vi "About WTI.vi"(0 "Description and Version":string, 1 "Designers":string[](array[string]), 2 "Contact Information In":string) -> ()   [LabVIEW 2019]
panel:
  in  "Exit":bool
  out "Project Description":string
  out "Designers:":string
  out "Contact Information:":string
  in  "SHDocVw.IWebBrowser2":refnum<k7>(container)
  # "System Developed with National Instruments LabVIEW"
  # "Copyright 2001 Wineman Technology Inc."
  # "Click Screen or Press Enter To Continue"
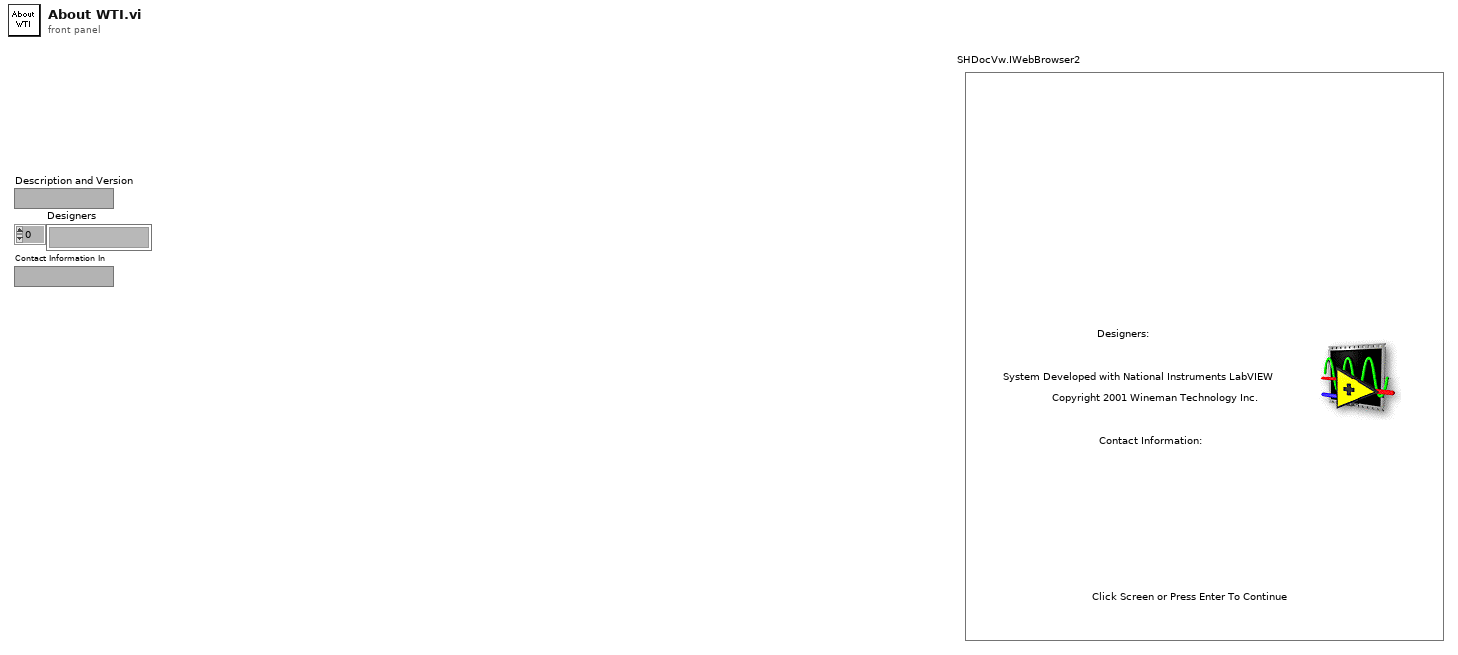
[diagram p1: front panel]
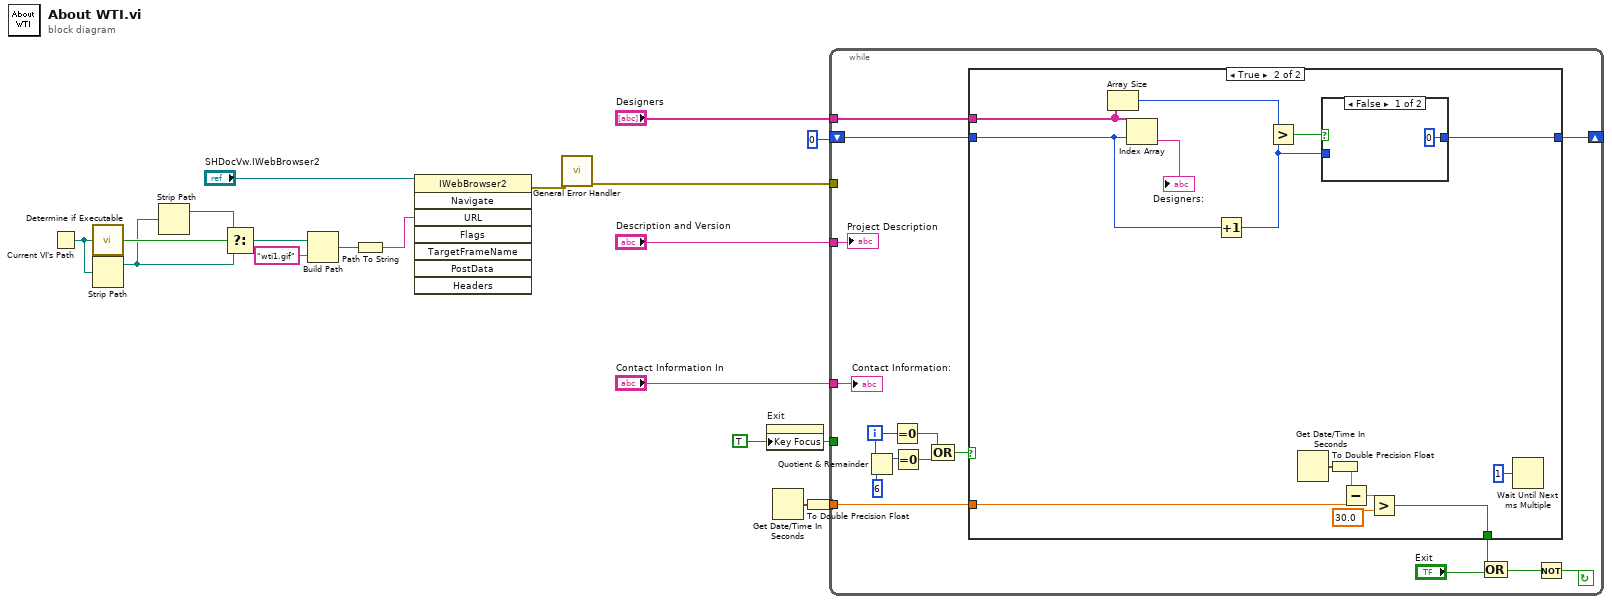
[diagram p0: block diagram]
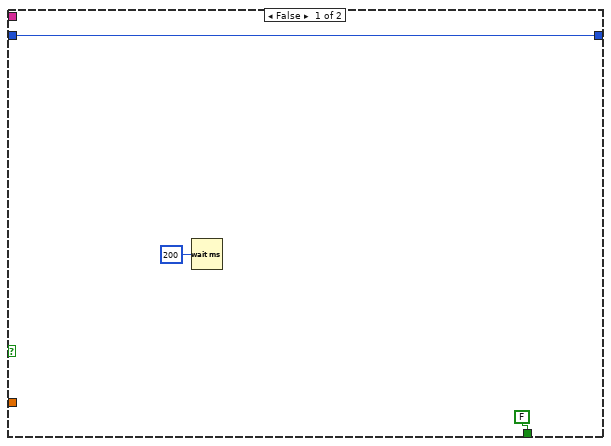
[diagram p2: hidden frame]
diagram:
  w13 = TRUE ("Key Focus")
  n1 = Current VI's Path() -> (path=w5:path)
  n2 = call "Determine if Executable.vi"("Path"=w5) -> ("EXE?"=w6:bool)
  n3 = Strip Path(path=w5) -> (stripped path=w4:path)  [unwired: 1 out]
  n4 = Strip Path(path=w4) -> (stripped path=w3:path)  [unwired: 1 out]
  n5 = Select(t=w3, s=w6, f=w4) -> (s? t:f=w2:path)
  n6 = Build Path(base path=w2, name or relative path="wti1.gif") -> (appended path=w11:path)
  n7 = Path To String(path=w11) -> (string=w10:string)
  n8 = invoke class="IWebBrowser2" method="Navigate"(reference="SHDocVw.IWebBrowser2", "URL"=w10) -> (error out=w9:errorcluster)  [unwired: 6 in, 7 out]
  n9 = call <vilib>:"General Error Handler.vi"("error in (no error)"=w9) -> ("error out"=w7:errorcluster)  [unwired: 10 in, 4 out]
  n10 = property on="Exit" class="Bool"("Key Focus"=w13) -> ()  [unwired: 2 in, 2 out]
  n11 = Get Date/Time In Seconds() -> (seconds since 1Jan1904=w1:timestamp)
  n12 = To Double Precision Float(number=w1) -> (double precision float=w18:dbl)
  n13 = while {
    tunnel: w7 -> [_]
    tunnel: w13 -> [_]
    tunnel: "Contact Information In" -> [w19]
    tunnel: "Description and Version" -> [w20]
    tunnel: "Designers" -> [w28]
    shift-left: 0 -> [w29]
    shift-right: [w21] -> _
    tunnel: w18 -> [w31]
    i -> [w27]
    stop <- w34 continue-if-true
    n14 = Quotient & Remainder(x=w27, y=6) -> (x-y*floor(x/y)=w24:i32)  [unwired: 1 out]
    n15 = Equal To 0?(x=w27) -> (x = 0?=w25:bool)
    n16 = Equal To 0?(x=w24) -> (x = 0?=w23:bool)
    n17 = Compound Arithmetic op=OR(w25, w23) -> (w22:bool)
    n18 = case shown="True" w22 {
      tunnel: w31 -> [_ w50]
      tunnel: [FALSE w47] -> w30
      tunnel: w29 -> [w36 w43]
      tunnel: w28 -> [_ w46]
      tunnel: [w36 w41] -> w21
      frame False {
        n19 = Wait (ms)(milliseconds to wait=u32 200) -> ()  [unwired: 1 out]
      }
      frame True {
        n20 = Array Size(array=w46) -> (size(s)=w44:i32)
        n21 = Index Array(array=w46, index=w43) -> (element=→"Designers:":string)
        n22 = Increment(x=w43) -> (x+1=w40:i32)
        n23 = Greater?(x=w44, y=w40) -> (0:w42:bool)
        n24 = Get Date/Time In Seconds() -> (seconds since 1Jan1904=w38:timestamp)
        n25 = case shown="False" w42 {
          tunnel: [0 w53] -> w41
          tunnel: w40 -> [_ w53]
          frame False {
          }
          frame True {
          }
        }
        n26 = To Double Precision Float(number=w38) -> (double precision float=w51:dbl)
        n27 = Subtract(x=w51, y=w50) -> (x-y=w49:dbl)
        n28 = Greater?(x=w49, y=30.0) -> (0:w47:bool)
        n29 = Wait Until Next ms Multiple(millisecond multiple=u32 1) -> ()  [unwired: 1 out]
      }
    }
    n30 = Compound Arithmetic op=OR(w30, "Exit") -> (w33:bool)
    n31 = Not(x=w33) -> (.not. x?=w34:bool)
    "Project Description" <- w20
    "Contact Information:" <- w19
  }
